vi "LVPortSetControlVariantValue.vi"(10 "Value":variant, 11 "ControlVariant":variant) -> (0 "IsControl":bool)   [LabVIEW 2017]
panel:
  out "Control being updated":string
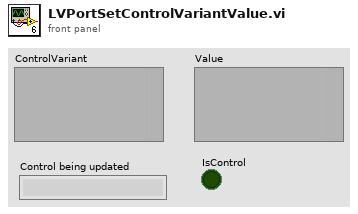
[diagram p1: front panel]
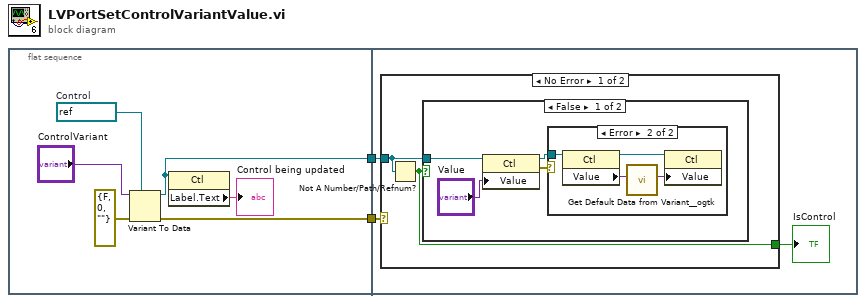
[diagram p0: block diagram]
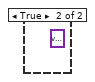
[diagram p3: hidden frame]
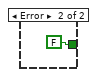
[diagram p4: hidden frame]
diagram:
  n1 = flat-sequence {
    tunnel: [w5] -> w2
    tunnel: [w4] -> w1
    tunnel: w2 -> [w10]
    tunnel: w1 -> [w9]
    frame #0 {
      w8 = refnum<vi> refnum  # Control
      n2 = Variant To Data(error in=errorcluster {"status"=FALSE, "code"=0, "source"=""}, type=w8, Variant="ControlVariant") -> (data=w4:refnum<vi>, error out=w5:errorcluster)
      n3 = property class="Ctl"(reference=w4) -> ("Label.Text"=→"Control being updated":string)  [unwired: 1 in, 2 out]
    }
    frame #1 {
      n4 = case shown="No Error" w10 {
        tunnel: w9 -> [w13 _]
        tunnel: [w12 FALSE] -> w11
        frame No Error {
          n5 = Not A Number/Path/Refnum?(number/path/refnum=w13) -> (NaN/Path/Refnum?=w12:bool)
          n6 = case shown="False" w12 {
            tunnel: w13 -> [w17 _]
            frame False {
              n7 = property class="Ctl"(reference=w17, "Value"="Value") -> (reference out=w14:refnum<vi>, error out=w15:errorcluster)  [unwired: 1 in]
              n8 = case shown="Error" w15 {
                tunnel: w14 -> [_ w21]
                frame No Error {
                }
                frame Error {
                  n9 = property class="Ctl"(reference=w21) -> (reference out=w18:refnum<vi>, "Value"=w20:variant)  [unwired: 1 in, 1 out]
                  n10 = call <userlib>:"Get Default Data from Variant__ogtk.vi"("Variant"=w20) -> ("Default VData"=w19:variant)  [unwired: 9 in, 1 out]
                  n11 = property class="Ctl"(reference=w18, "Value"=w19) -> ()  [unwired: 1 in, 2 out]
                }
              }
            }
            frame True {
              (unwired) variant ("Value")
            }
          }
        }
        frame Error {
        }
      }
      "IsControl" <- w11
    }
  }
